vi "Initialise.vi"(8 "error in (no error)":errorcluster, 10 "Message in":refnum<class "InitialiseMessage.lvclass">, 11 "Waveform in":refnum<class "Waveform.lvclass">) -> (0 "error out":errorcluster, 3 "Waveform out":refnum<class "Waveform.lvclass">)   [LabVIEW 2012, in "Waveform.lvclass"]
doc: "This method is called when an initialise message is received. It mainly initialises the RabbitMQ connectivity. \n\nOverride this method when your component needs special initialisation (e.g. of software or hardware resources). In that case, don't forget to call the parent for proper implementation. If your component owns subcomponents, they count as resources, so you have to initialise them by calling their own initialise functions"
uses:
  Waveform.lvclass
  <vilib>/Distrio/Murmex/InitialiseMessage/InitialiseMessage.lvclass
  <vilib>/Distrio/Murmex/Murmex/Murmex.lvclass
  Waveform.lvclass/Waveform.ctl
panel:
  # "This method is called when the INTIALISE\ntrigger is sent. \n\nOverride this method when your component needs to\nrespond to this trigger. \n\nCall parent for proper implementation"
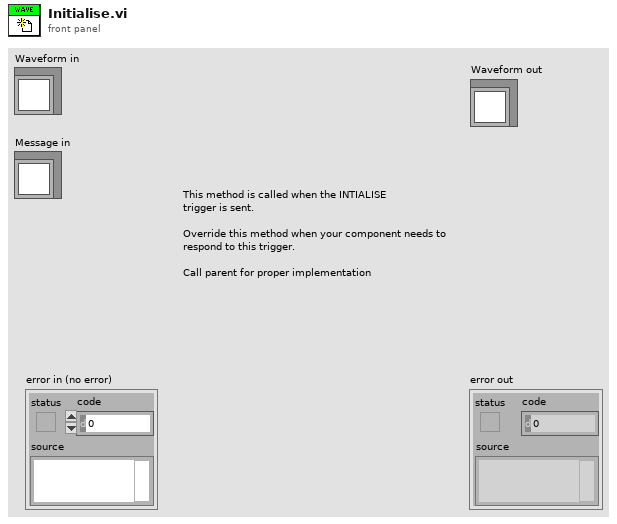
[diagram p1: front panel]
types:
  T1 = enum8{"Enabled", "Disabled", "Disabled and Grayed Out"}
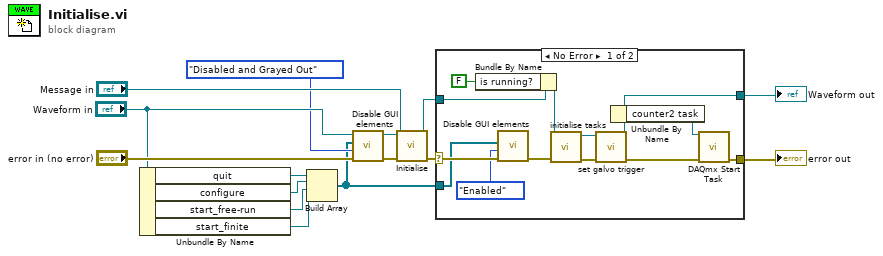
[diagram p0: block diagram]
diagram:
  n1 = Unbundle By Name("Waveform in") -> ("quit"=w8:refnum<vi>, "configure"=w7:refnum<vi>, "start_free-run"=w6:refnum<vi>, "start_finite"=w5:refnum<vi>)
  n2 = Build Array(w8, w7, w6, w5) -> (w3:refnum<vi>[])
  n3 = call <vilib>:"Disable GUI elements.vi"("error in (no error)"="error in (no error)", "enabled state"=T1."Disabled and Grayed Out", "control refs"=w3) -> ("error out"=w10:errorcluster)  [unwired: 8 in]
  n4 = call-parent "Initialise.vi"("error in (no error)"=w10, "Message in"="Message in", "Murmex in"="Waveform in") -> ("error out"=w1:errorcluster, "Murmex out"=w2:refnum<class "Waveform.lvclass">)  [unwired: 7 in]
  n5 = case shown="No Error" w1 {
    selector: w1 -> [w27 w28]
    tunnel: w2 -> [w23 w29]
    tunnel: [w17 w28] -> w13
    tunnel: [w16 w29] -> w12
    tunnel: w3 -> [w24 _]
    frame No Error {
      n6 = Bundle By Name(cluster=w23, "is running?"=FALSE ("runtime.is running?")) -> (w22:refnum<class "Waveform.lvclass">)
      n7 = call <vilib>:"Disable GUI elements.vi"("error in (no error)"=w27, "enabled state"=T1."Enabled", "control refs"=w24) -> ("error out"=w26:errorcluster)  [unwired: 8 in]
      n8 = call-dynamic "initialise tasks.vi"("error in (no error)"=w26, "Waveform in"=w22) -> ("error out"=w19:errorcluster, "Waveform out"=w20:refnum<class "Waveform.lvclass">)  [unwired: 8 in]
      n9 = call-dynamic "set galvo trigger.vi"("error in (no error)"=w19, "Waveform in"=w20) -> ("error out"=w18:errorcluster, "Waveform out"=w16:refnum<class "Waveform.lvclass">)  [unwired: 8 in]
      n10 = Unbundle By Name(w16) -> ("counter2 task"=w15:refnum<k21>)
      n11 = call <vilib>:"DAQmx Start Task.vi"("task/channels in"=w15, "error in"=w18) -> ("error out"=w17:errorcluster)  [unwired: 12 in, 1 out]
    }
    frame Error {
    }
  }
  "error out" <- w13
  "Waveform out" <- w12
